vi "LV to DAT.vi"(6 "append to file? (new file:F)":bool, 7 "path":path, 8 "wavenames (.Vx, etc)":string[](array[string]), 9 "Data":string[](array[string]), 10 "Comments":string, 11 "filename":string) -> (3 "new file path (Not A Path if cancelled)":path)   [LabVIEW 2013]
uses:
  <vilib>/Utility/file.llb/Write To Spreadsheet File (string).vi
panel:
  out "appended array":string[][](array[string])
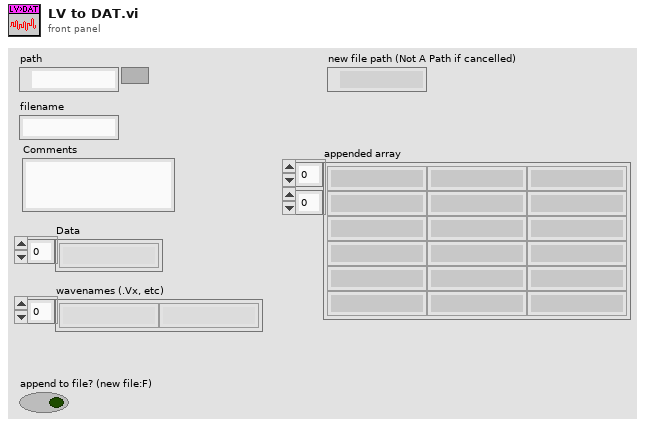
[diagram p1: front panel]
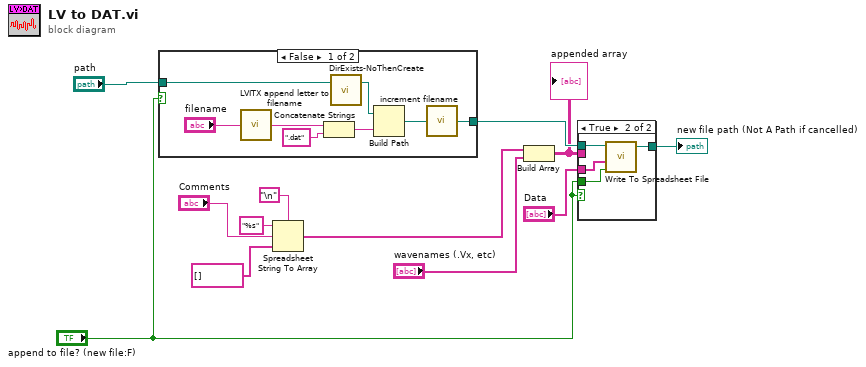
[diagram p0: block diagram]
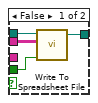
[diagram p3: hidden frame]
diagram:
  n1 = case shown="False" "append to file? (new file:F)" {
    tunnel: [w20 w21] -> w12
    tunnel: "path" -> [w18 w21]
    frame False {
      n2 = call <userlib>:"LVITX append letter to filename.vi"("string in"="filename") -> ("string out"=w13:string)
      n3 = Concatenate Strings(w13, ".dat" ("string")) -> (w14:string)
      n4 = call <userlib>:"DirExists-NoThenCreate.vi"("path"=w18) -> ("created path"=w15:path)  [unwired: 1 in, 1 out]
      n5 = Build Path(base path=w15, name or relative path=w14) -> (appended path=w16:path)
      n6 = call <userlib>:"increment filename.vi"("path"=w16) -> ("modified path"=w20:path)
    }
    frame True {
    }
  }
  n7 = Spreadsheet String To Array(delimiter (Tab)="\n", format string="%s", spreadsheet string="Comments", array type (2D Dbl)=string[] []) -> (array=w4:string[])
  n8 = Build Array(w4, "wavenames (.Vx, etc)") -> (w7:string[][])
  "appended array" <- w7
  n9 = case shown="True" "append to file? (new file:F)" {
    tunnel: "append to file? (new file:F)" -> [w25 w29]
    tunnel: w7 -> [w24 _]
    tunnel: [w23 w28] -> w9
    tunnel: "Data" -> [_ w26]
    tunnel: w12 -> [w22 w27]
    frame False {
      n10 = call-poly <vilib>:"Write To Spreadsheet File.vi"("append to file? (new file:F)"=w25, "2D data"=w24, "file path (dialog if empty)"=w22) -> ("new file path (Not A Path if cancelled)"=w23:path)  [unwired: 5 in]
    }
    frame True {
      n11 = call-poly <vilib>:"Write To Spreadsheet File.vi"("append to file? (new file:F)"=w29, "1D data"=w26, "file path (dialog if empty)"=w27) -> ("new file path (Not A Path if cancelled)"=w28:path)  [unwired: 5 in]
    }
  }
  "new file path (Not A Path if cancelled)" <- w9
